vi "BLE Channel Number to Frequency.vi"(8 "error in (no error)":errorcluster, 11 "BLE  Channel":u8) -> (0 "error out":errorcluster, 3 "Frequency, Hz":dbl)   [LabVIEW 2026, in "Nordic nRF52 DK DTM Test.lvlib"]
uses:
  Nordic nRF52 DK DTM Test.lvlib
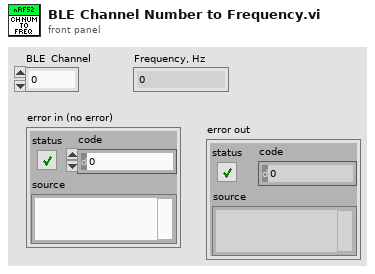
[diagram p1: front panel]
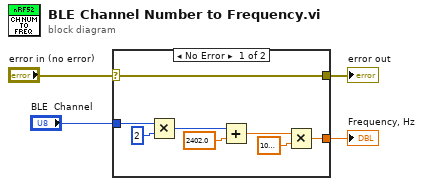
[diagram p0: block diagram]
diagram:
  n1 = case shown="No Error" "error in (no error)" {
    selector: "error in (no error)" -> [w5 w13]
    tunnel: [w12 _] -> w4
    tunnel: "BLE  Channel" -> [w8 _]
    tunnel: [w5 w13] -> w1
    frame No Error {
      n2 = Multiply(x=w8, y=u16 2) -> (x*y=w7:u16)
      n3 = Add(x=w7, y=2402.0) -> (x+y=w10:dbl)
      n4 = Multiply(x=w10, y=1000000.0) -> (x*y=w12:dbl)
    }
    frame Error {
    }
  }
  "Frequency, Hz" <- w4
  "error out" <- w1
